vi "SCMP - Cbk end sound.vi"(10 "duration (msec)":u32=1000, 11 "frequency (Hz)":u32=700) -> ()   [LabVIEW 2014]
panel:
  in  "duration (msec) 2":u32=1000
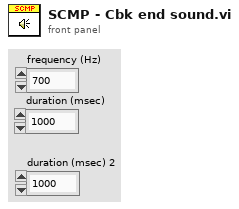
[diagram p1: front panel]
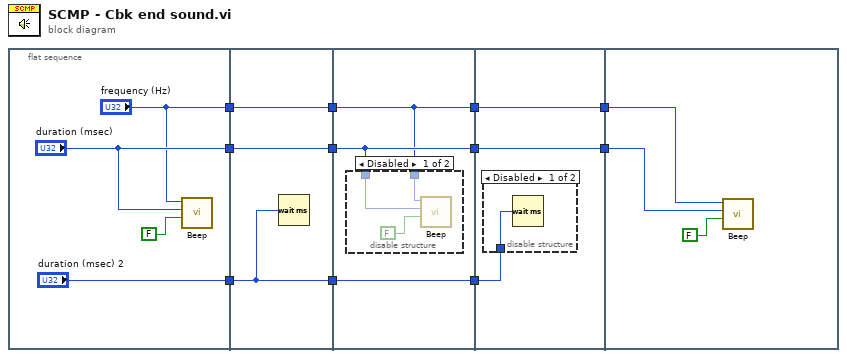
[diagram p0: block diagram]
diagram:
  n1 = flat-sequence {
    tunnel: ["duration (msec)"] -> w11
    tunnel: ["frequency (Hz)"] -> w9
    tunnel: ["duration (msec) 2"] -> w3
    tunnel: w11 -> [w18]
    tunnel: [w18] -> w10
    tunnel: w9 -> [w17]
    tunnel: [w17] -> w8
    tunnel: w3 -> [w16]
    tunnel: [w16] -> w2
    tunnel: w10 -> [w21]
    tunnel: w8 -> [w20]
    tunnel: [w21] -> w7
    tunnel: [w20] -> w5
    tunnel: w2 -> [w19]
    tunnel: [w19] -> w1
    tunnel: w7 -> [w27]
    tunnel: [w27] -> w6
    tunnel: w5 -> [w26]
    tunnel: [w26] -> w4
    tunnel: w1 -> [w25]
    tunnel: w6 -> [w29]
    tunnel: w4 -> [w30]
    frame #0 {
      n2 = call <vilib>:"Beep.vi"("use system alert? (T)"=FALSE, "duration (msec)"="duration (msec)", "frequency (Hz)"="frequency (Hz)") -> ()  [unwired: 9 in]
    }
    frame #1 {
      n3 = Wait (ms)(milliseconds to wait=w16) -> ()  [unwired: 1 out]
    }
    frame #2 {
      n4 = disable-structure shown="Disabled" {
        disable-tunnel: w21 -> [w23 _]
        disable-tunnel: w20 -> [w22 _]
        frame Disabled {
          n5 = call <vilib>:"Beep.vi"("use system alert? (T)"=FALSE, "duration (msec)"=w23, "frequency (Hz)"=w22) -> ()  [unwired: 9 in]
        }
        frame Enabled {
        }
      }
    }
    frame #3 {
      n6 = disable-structure shown="Disabled" {
        disable-tunnel: w25 -> [w28 _]
        frame Disabled {
          n7 = Wait (ms)(milliseconds to wait=w28) -> ()  [unwired: 1 out]
        }
        frame Enabled {
        }
      }
    }
    frame #4 {
      n8 = call <vilib>:"Beep.vi"("use system alert? (T)"=FALSE, "duration (msec)"=w29, "frequency (Hz)"=w30) -> ()  [unwired: 9 in]
    }
  }
